vi "Status_change.vi"(1 "Routing":bool=TRUE, 3 "OP10B STATUS":i32) -> (0 "Status Change":bool)   [LabVIEW 2020]
uses:
  <userlib>/_OpenG.lib/comparison/comparison.llb/I32 Changed__ogtk.vi
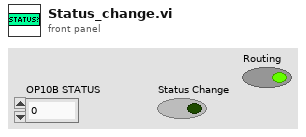
[diagram p1: front panel]
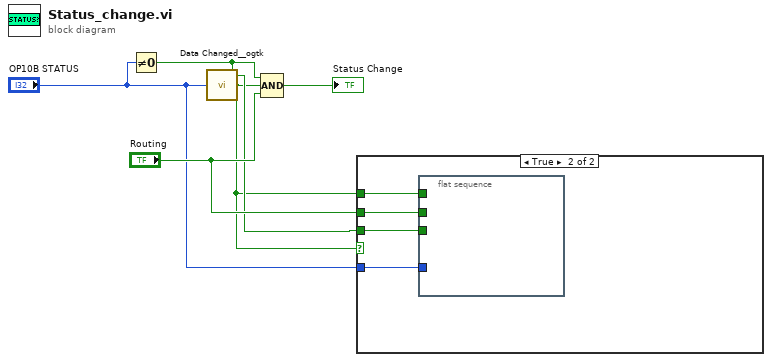
[diagram p0: block diagram]
diagram:
  n1 = Not Equal To 0?(x="OP10B STATUS") -> (x != 0?=w3:bool)
  n2 = call-poly <userlib>:"Data Changed__ogtk.vi"("I32"="OP10B STATUS") -> ("Changed"=w2:bool)
  n3 = Compound Arithmetic op=AND(w3, w2, "Routing") -> (→"Status Change":bool)
  n4 = case shown="True" w2 {
    tunnel: "Routing" -> [_ w8]
    tunnel: w3 -> [_ w9]
    tunnel: w2 -> [_ w7]
    tunnel: "OP10B STATUS" -> [_ w6]
    frame False {
    }
    frame True {
      n5 = flat-sequence {
        tunnel: w9 -> [_]
        tunnel: w8 -> [_]
        tunnel: w7 -> [_]
        tunnel: w6 -> [_]
        frame #0 {
        }
      }
    }
  }
